vi "ArmControlCalibrate.vi"() -> ()   [LabVIEW 2015]
uses:
  <vilib>/Rock Robotics/WPI/CAN/TalonSRX/WPI_CANTalonSRX_APIFeedbackSelect.ctl
  <vilib>/Rock Robotics/WPI/CAN/TalonSRX/WPI_CANTalonSRX_APIControlMode.ctl
  <vilib>/Rock Robotics/WPI/Joystick/WPI_JoystickDeviceEnum.ctl
  <vilib>/Platform/TimedLoop/XDataNode/timing_clust.ctl
  <vilib>/Platform/TimedLoop/XDataNode/nitl_modes.ctl
  <vilib>/Platform/TimedLoop/XDataNode/wakeup.ctl
  <vilib>/Rock Robotics/WPI/MotorControl/WPI_MotorControlOpenCANTalonSRX.vi
  Team900-VIs/Logitech/F510/F510-X.vi
  <vilib>/addons/control/pid/pid.llb/PID Control Input Filter (DBL).vi
  <vilib>/addons/control/pid/pid.llb/PID (DBL).vi
  Robot Global Data.vi
  <vilib>/Utility/config.llb/Read Key (Double).vi
  <vilib>/Utility/config.llb/Write Key (Double).vi
  <vilib>/Platform/TimedLoop/XDataNode/XDataNode.xnode
  <vilib>/Platform/TimedLoop/XDataNode/XDNodeRunTimeDep.lvlib
  <vilib>/Utility/config.llb/NI_LVConfig.lvlib
  Team900-VIs/Team900SwerveDrive/Team900SwerveDrive.lvlib
  <vilib>/addons/control/pid/NI_PID_pid.lvlib
panel:
  in  "Motor to set offset":enum16{"Pivot", "Wrist", "Claw"}(ring)
  in  "Set":bool
  in  "stop":bool
  in  "Mode":enum32{"Manual Mode", "PID Tuning"}(tab)
  out "(manual) error out":errorcluster
  out "Sensor Position \n(manual) (offset)":dbl
  in  "Control this motor":enum16{"Pivot", "Extension", "Wrist", "Claw"}(ring)
  in  "Max %Vbus":dbl=0.1 format="%#_13g"
  out "Forward Limit Switch Closed":bool
  out "Reverse Limit Switch Closed":bool
  out "Applied Throttle (manual)":dbl
  out "raw sensor position":dbl
  out "Pivot Offset":dbl
  out "Claw Offset (m)":dbl
  out "Wrist Offset":dbl
  out "analog in chart":dbl(graph)
  in  "NI PID":bool
  in  "Setpoint":T1
  in  "Enable":T2
  in  "Motor Controller":enum16{"Pivot", "Extension", "Wrist"}(ring)
  in  "PID":cluster{"P":dbl, "I":dbl, "D":dbl}
  out "error out":errorcluster
  in  "Set":bool=TRUE
  in  "Ramp Rate":dbl
  out "Applied Throttle":dbl
  out "Encoder Position":dbl
  out "Analog In":dbl
  out "Sensor Position":dbl
  out "Difference":dbl
  out "Waveform Chart":cluster{"Pivot":dbl, "Sensor Position":dbl, dbl}(graph)
  out "Angle":dbl(knob) scale=3.14159..-3.14159
  out "Extension":dbl(slide) scale=0.0..100.0
  in  "Claw":bool
  in  "output range":cluster{"output high":dbl, "output low":dbl}={"output high"=100.0, "output low"=-100.0} {"output low" format="%.2f"; "output high" format="%.2f"}
  in  "PID gains":T3={"proportional gain (Kc)"=1.0, "integral time (Ti, min)"=0.0, "derivative time (Td, min)"=0.0} {"derivative time (Td, min)" format="%.3f"; "integral time (Ti, min)" format="%.3f"; "proportional gain (Kc)" format="%.3f"}
  # "360 Ticks on extension"
  # "Left Stick controls whatever motor is selected"
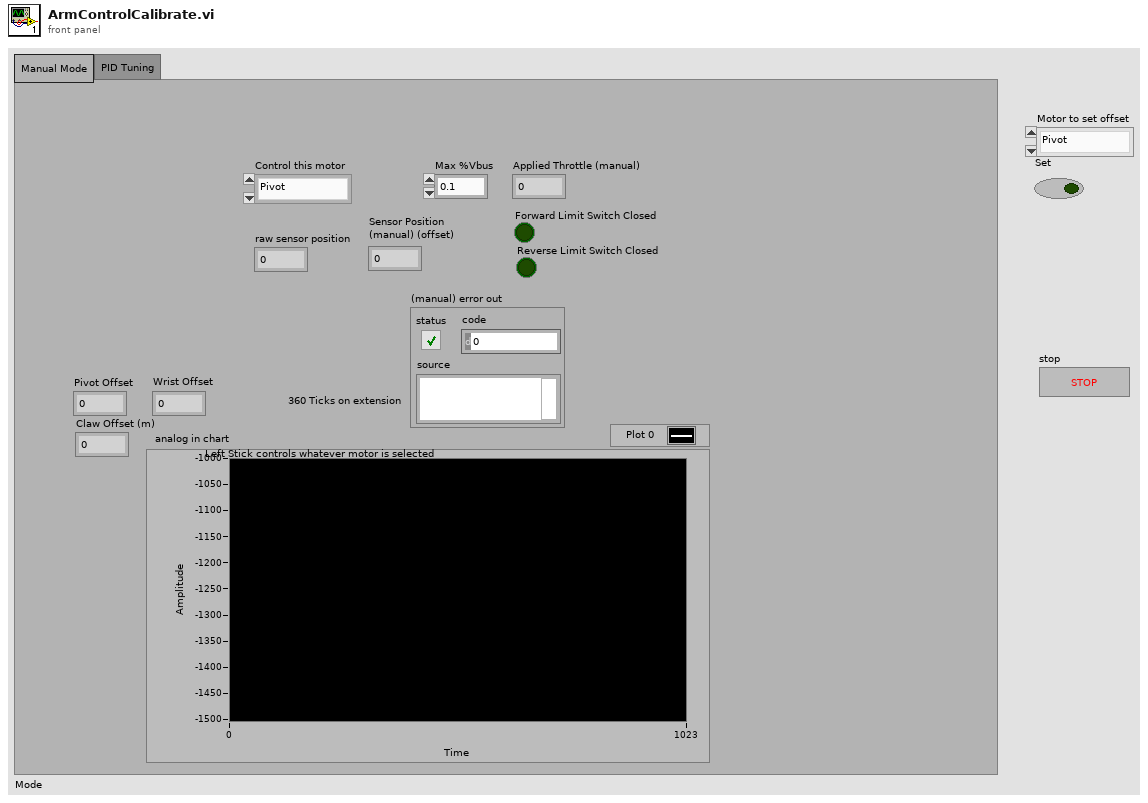
[diagram p1: front panel]
types:
  T1 = cluster{"Pivot":dbl, "Extension":dbl, "Wrist":dbl}
  T2 = cluster{"Pivot":bool, "Exension":bool, "Wrist":bool}
  T3 = cluster{"proportional gain (Kc)":dbl, "integral time (Ti, min)":dbl, "derivative time (Td, min)":dbl}
  T4 = typedef "WPI_CANTalonSRX_APIFeedbackSelect.ctl" = enum16{"Digital Quadrature Encoder", "Analog Potentiometer", "Analog Encoder"}
  T5 = cluster{"Feedback Sensor":T4, "Device Number":u8, "Invert Motor":bool, "Reverse Sensor":bool}
  T6 = typedef "WPI_CANTalonSRX_APIControlMode.ctl" = enum8{"Percent VBus", "Speed", "Position", "Slave", "Unchanged / Invalid"}
  T7 = typedef "NI_LVConfig.lvlib/Config Data RefNum.ctl" = refnum<k1>
  T8 = cluster{"Feedback Sensor":T4, "Device Number":u8, "Invert Motor":bool, "Reverse Sensor":bool}[]
  T9 = typedef "WPI_MotorControlDeviceRef.ctl" = cluster{"DeviceStatus":errorcluster, "Type":T10, "PWM":cluster{"PWM Channel":T11, "DeadBand":T12}, "CAN":cluster{"Device Number":u8, "Control Mode":T13, "Semaphore":T14, "Max Vout":dbl, "TalonSRX Control Mode":T6}, "Invert":bool, "TransformRef":T15, "InvTransformRef":T15}
  T10 = typedef "WPI_MotorControlType.ctl" = enum16{"PWM", "CAN", "CANTalonSRX"}
  T11 = typedef "FPGA_DIOPWMChannel.ctl" = enum8{"PWM 0", "PWM 1", "PWM 2", "PWM 3", "PWM 4", "PWM 5", "PWM 6", "PWM 7", "PWM 8", "PWM 9", "PWM MXP 0", "PWM MXP 1", "PWM MXP 2", "PWM MXP 3", "PWM MXP 4", "PWM MXP 5", "PWM MXP 6", "PWM MXP 7", "PWM MXP 8", "PWM MXP 9", "Invalid"}
  T12 = typedef "WPI_PWMDeadband.ctl" = cluster{"Name":string, "maxPositivePwm":i32, "minPositivePwm":i32, "centerPwm":i32, "maxNegativePwm":i32, "minNegativePwm":i32, "angularRange":u16}
  T13 = typedef "WPI_CANJaguar_ControlMode.ctl" = enum8{"Percent VBus", "Current", "Speed", "Position", "Voltage"}
  T14 = typedef "Semaphore RefNum" = refnum<k1>
  T15 = typedef "WPI_PWMTransform_ConPane.ctl" = refnum<vi>
  T16 = typedef "WPI_CANTalonSRX_GlobalStatus.ctl" = cluster{"Applied Throttle":dbl, "Module Enabled":bool, "CAN Error":errorcluster, "Closed Loop Error":dbl, "Forward Limit Switch Closed":bool, "Reverse Limit Switch Closed":bool, "Sensor Position":dbl, "Sensor Velocity":dbl, "Current":dbl, "Sticky Fault - Over Temp":bool, "Sticky Fault - Under Voltage":bool, "Sticky Fault - Forward Limit":bool, "Sticky Fault - Reverse Limit":bool, "Sticky Fault - Forward Soft Limit":bool, "Sticky Fault - Reverse Soft Limit":bool, "Brake is Enabled":bool, "Encoder Position":dbl, "Encoder Velocity":dbl, "Encoder Index Count":dbl, "Encoder A Pin State":bool, "Encoder B Pin State":bool, "Encoder Index Pin State":bool, "Analog In":dbl, "Analog In Velocity":dbl, "Temperature (C)":dbl, "Battery Voltage":dbl}
  T17 = typedef "WPI_JoystickDeviceEnum.ctl" = enum16{"USB 0", "USB 1", "USB 2", "USB 3", "USB 4", "USB 5"}
  T18 = enum16{"Open", "Close", "Continue", "Stop", "Toggle"}
  T19 = typedef "XDNodeRunTimeDep.lvlib/timing_clust.ctl" = cluster{"Expected End [f-1]":u64, "Actual End [f-1]":u64, "Finished Late? [f-1]":bool, "Expected End [i-1]":u64, "Actual End [i-1]":u64, "Finished Late? [i-1]":bool, "Expected Start [i]":u64, "Actual Start [i]":u64, "Expected Start [f]":u64, "Actual Start [f]":u64, "Source Name":string, "Structure Name":string, "Period":i64, "Deadline":i64, "Offset":i64, "Start":i64, "Priority":i32, "Timeout":i32, "Mode":T20, "Wakeup Reason":T21, "Error":errorcluster, "Source Type":string, "Secondary Source Type":string, "Global End Time":u64, "Global Start Time":u64, "Frame Duration":u64, "Iteration Duration":u64, "Assigned CPU":i32, "I/O Scan Engine Mode":u32}
  T20 = typedef "XDNodeRunTimeDep.lvlib/nitl_modes.ctl" = enum32{"No Change", "Process missed periods, maintain original phase", "Discard missed periods, maintain original phase", "Process missed periods, ignore original phase", "Discard missed periods, ignore original phase"}
  T21 = typedef "XDNodeRunTimeDep.lvlib/wakeup.ctl" = enum32{"Normal", "Aborted", "Asynchronous wakeup", "Timing source error", "Timed loop error", "Timeout"}
  T22 = typedef "WPI_JoystickDevRef.ctl" = cluster{"Device":T17}
  T23 = cluster{"Applied Throttle":dbl, "Encoder Position":dbl, "Sensor Position":dbl, "Analog In":dbl}
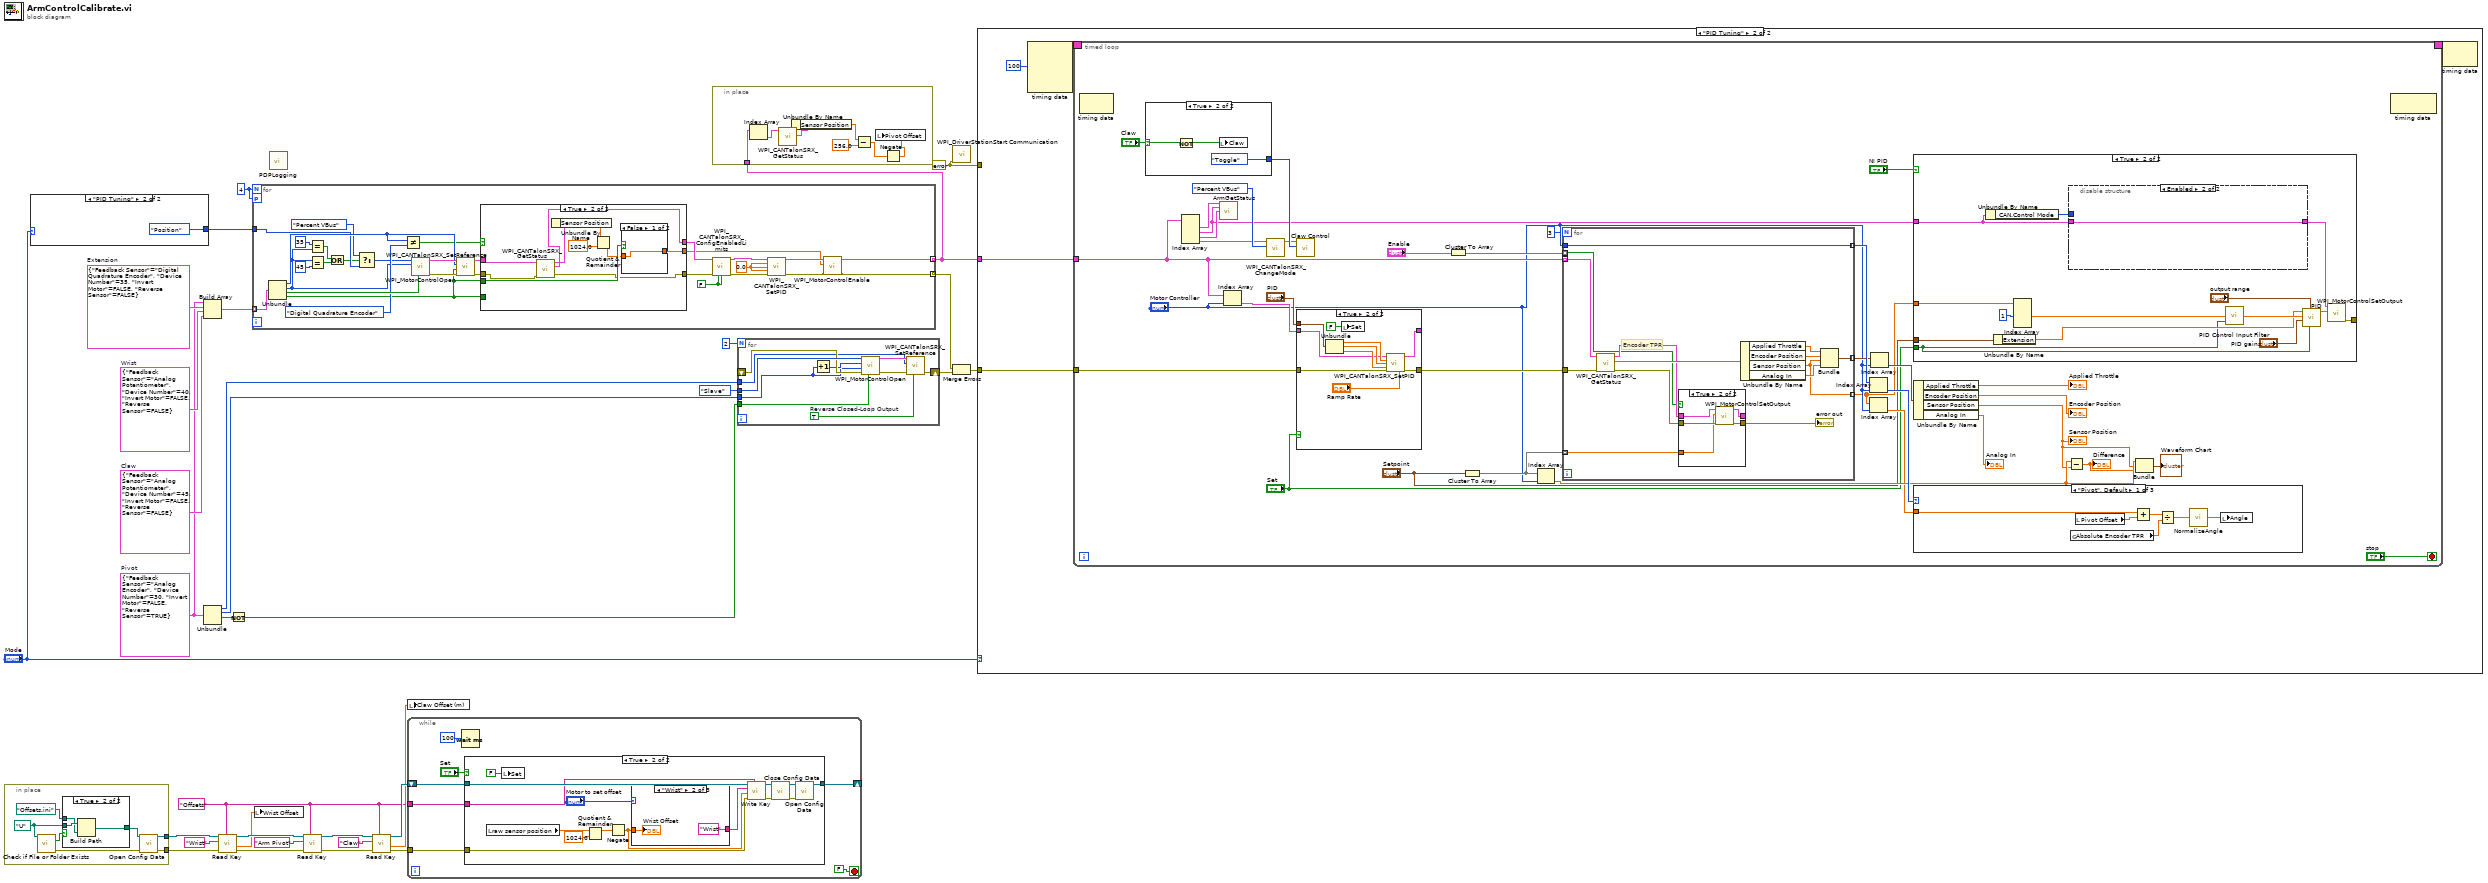
[diagram p0: block diagram]
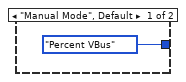
[diagram p2: hidden frame]
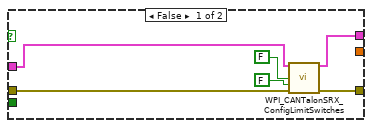
[diagram p3: hidden frame]
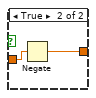
[diagram p4: hidden frame]
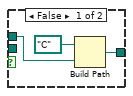
[diagram p5: hidden frame]
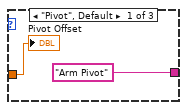
[diagram p7: hidden frame]
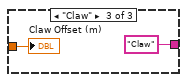
[diagram p8: hidden frame]
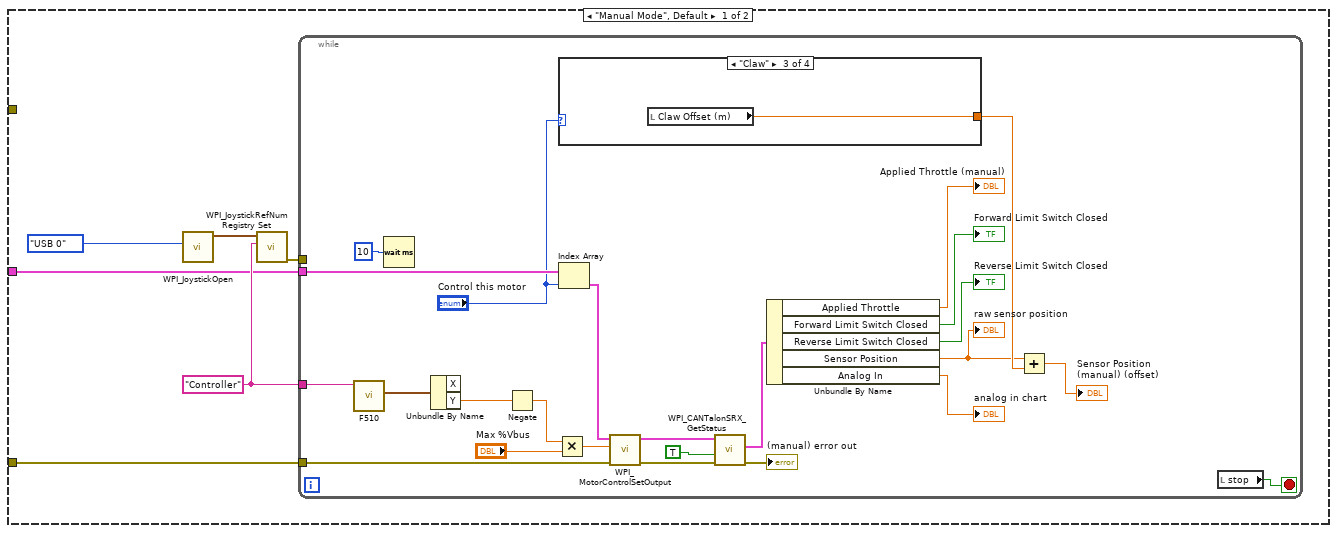
[diagram p9: hidden frame]
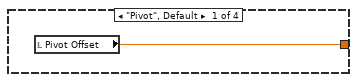
[diagram p10: hidden frame]
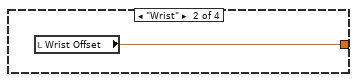
[diagram p11: hidden frame]
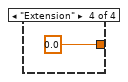
[diagram p12: hidden frame]
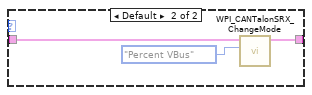
[diagram p15: hidden frame]
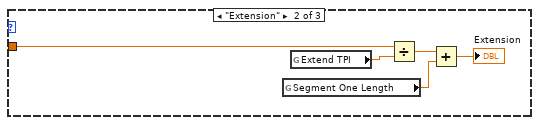
[diagram p16: hidden frame]
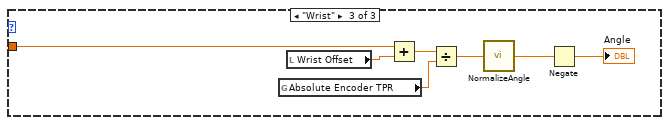
[diagram p17: hidden frame]
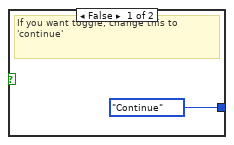
[diagram p19: hidden frame]
diagram:
  w2 = T5 {"Feedback Sensor"=enum."Analog Encoder", "Device Number"=30, "Invert Motor"=FALSE, "Reverse Sensor"=TRUE}  # Pivot
  w3 = T5 {"Feedback Sensor"=enum."Digital Quadrature Encoder", "Device Number"=35, "Invert Motor"=FALSE, "Reverse Sensor"=FALSE}  # Extension
  w16 = 4
  w19 = "Offsets" ("section")
  w17 = T5 {"Feedback Sensor"=enum."Analog Potentiometer", "Device Number"=45, "Invert Motor"=FALSE, "Reverse Sensor"=FALSE}  # Claw
  w18 = T5 {"Feedback Sensor"=enum."Analog Potentiometer", "Device Number"=40, "Invert Motor"=FALSE, "Reverse Sensor"=FALSE}  # Wrist
  w33 = errorcluster {"status"=FALSE, "code"=0, "source"=""} ("error constant")
  n1 = in-place {
    in-place-border: [w39] -> w32
    in-place-border: [w38] -> w31
    w34 = path "U:/" ("base path")
    n2 = call <vilib>:"Check if File or Folder Exists.vi"("path"=w34) -> ("error out"=w40:errorcluster, "file or folder exists?"=w35:bool)  [unwired: 8 in, 1 out]
    n3 = case shown="True" w35 {
      tunnel: path "Offsets.ini" ("default name") -> [w43 w44]
      tunnel: [w42 w45] -> w37
      tunnel: w34 -> [_ w46]
      frame False {
        n4 = Build Path(base path=path "C:/", name or relative path=w43) -> (appended path=w42:path)
      }
      frame True {
        n5 = Build Path(base path=w46, name or relative path=w44) -> (appended path=w45:path)
      }
    }
    n6 = call <vilib>:"Open Config Data.vi"("error in (no error)"=w40, "configuration file path"=w37) -> ("error out"=w39:errorcluster, "refnum"=w38:T7)  [unwired: 1 in, 7 out]
  }
  n7 = case shown="\"PID Tuning\"" "Mode" {
    tunnel: [WPI_CANTalonSRX_APIControlMode."Percent VBus" ("Control Mode") WPI_CANTalonSRX_APIControlMode."Position" ("Control Mode")] -> w12
    frame "Manual Mode", Default {
    }
    frame "PID Tuning" {
    }
  }
  n8 = Build Array(w2, w3, w18, w17) -> (w15:T8)
  n9 = Unbundle(w2) -> ("Feedback Sensor"=w8:T4, "Device Number"=w9:u8, "Invert Motor"=w6:bool)  [unwired: 1 out]
  n10 = call-poly <vilib>:"Read Key.vi"("section"=w19, "error in (no error)"=w32, "key"="Wrist", "refnum"=w31) -> ("error out"=w27:errorcluster, "value"=w21:dbl, "refnum out"=w30:T7)  [unwired: 4 in, 1 out]
  n11 = Not(x=w6) -> (.not. x?=w7:bool)
  n12 = for {
    N: w16 -> [_]
    workers-P: w16 -> [_]
    tunnel: [w51] -> w1 mode=indexing
    tunnel: [w52] -> w14 mode=indexing
    tunnel: w15 -> [w76] mode=indexing
    tunnel: w12 -> [w66]
    w55 = FALSE
    w70 = 0.0
    n13 = Unbundle(w76) -> ("Feedback Sensor"=w72:T4, "Device Number"=w62:u8, "Invert Motor"=w75:bool, "Reverse Sensor"=w50:bool)
    n14 = Equal?(x=u8 35, y=w62) -> (x = y?=w64:bool)
    n15 = Equal?(x=w62, y=u8 45) -> (x = y?=w63:bool)
    n16 = Or(x=w64, y=w63) -> (x .or. y?=w65:bool)
    n17 = Select(t=WPI_CANTalonSRX_APIControlMode."Percent VBus" ("f"), s=w65, f=w66) -> (s? t:f=w68:T6)
    n18 = Not Equal?(x=w72, y=WPI_CANTalonSRX_APIFeedbackSelect."Digital Quadrature Encoder") -> (x != y?=w69:bool)
    n19 = call-poly <vilib>:"WPI_MotorControlOpen.vi"("Invert"=w75, "Device Number"=w62, "Control Mode"=w68) -> ("error out"=w78:errorcluster, "MotorControlDeviceRef"=w77:T9)  [unwired: 7 in]
    n20 = call <vilib>:"WPI_CANTalonSRX_SetReference.vi"("error in (no error)"=w78, "Reverse Feedback Sensor"=w50, "Feedback Reference"=w72, "CAN Talon SRX Ref"=w77) -> ("error out"=w74:errorcluster, "CAN Talon SRX Ref"=w73:T9)  [unwired: 6 in]
    n21 = case shown="True" w69 {
      tunnel: w50 -> [_ _]
      tunnel: w74 -> [w79 w92]
      tunnel: w73 -> [w80 w93]
      tunnel: [w84 w88] -> w59
      tunnel: [w83 w87] -> w58
      tunnel: w50 -> [_ w91]
      tunnel: [_ w89] -> w49
      frame False {
        n22 = call <vilib>:"WPI_CANTalonSRX_ConfigLimitSwitches.vi"("CAN Talon SRX Ref"=w80, "Forward Limit Switch Normally Open"=FALSE, "Reverse Limit Switch Normally Open"=FALSE, "error in (no error)"=w79) -> ("CAN Talon SRX Ref"=w84:T9, "error out"=w83:errorcluster)  [unwired: 10 in]
      }
      frame True {
        n23 = call <vilib>:"WPI_CANTalonSRX_GetStatus.vi"("error in (no error)"=w92, "CAN Talon SRX Ref"=w93) -> ("error out"=w87:errorcluster, "Talon SRX Status"=w94:T16, "CAN Talon SRX Ref"=w88:T9)  [unwired: 7 in]
        n24 = Unbundle By Name(w94) -> ("Sensor Position"=w90:dbl)
        n25 = Quotient & Remainder(x=w90, y=1024.0) -> (floor(x/y)=w86:dbl)  [unwired: 1 out]
        n26 = case shown="False" w91 {
          tunnel: w86 -> [w95 w97]
          tunnel: [w95 w96] -> w89
          frame False {
          }
          frame True {
            n27 = Negate(x=w97) -> (-x=w96:dbl)
          }
        }
      }
    }
    n28 = call <vilib>:"WPI_CANTalonSRX_ConfigEnabledLimits.vi"("CAN Talon SRX Ref"=w59, "error in (no error)"=w58, "Forward Soft Limit Enable"=w55, "Reverse Soft Limit Enable"=w55) -> ("CAN Talon SRX Ref"=w57:T9, "error out"=w56:errorcluster)  [unwired: 10 in]
    n29 = call <vilib>:"WPI_CANTalonSRX_SetPID.vi"("CAN Talon SRX Ref"=w57, "P"=w70, "I"=w70, "D"=w70, "error in (no error)"=w56) -> ("CAN Talon SRX Ref Out"=w54:T9, "error out"=w53:errorcluster)  [unwired: 9 in]
    n30 = call <vilib>:"WPI_MotorControlEnable.vi"("error in (no error)"=w53, "Encoder Initial Position"=w49, "CAN Jaguar Ref"=w54) -> ("error out"=w52:errorcluster, "CAN Jaguar Ref"=w51:T9)  [unwired: 7 in]
  }
  n31 = local write "Wrist Offset"(w21) -> ()
  n32 = call "PDPLogging.vi"() -> ()  [unwired: 12 in]
  n33 = call-poly <vilib>:"Read Key.vi"("section"=w19, "error in (no error)"=w27, "key"="Arm Pivot", "refnum"=w30) -> ("error out"=w26:errorcluster, "refnum out"=w29:T7)  [unwired: 4 in, 2 out]
  n34 = call-poly <vilib>:"Read Key.vi"("section"=w19, "error in (no error)"=w26, "key"="Claw", "refnum"=w29) -> ("error out"=w25:errorcluster, "value"=w20:dbl, "refnum out"=w28:T7)  [unwired: 4 in, 1 out]
  n35 = local write "Claw Offset (m)"(w20) -> ()
  n36 = while {
    tunnel: w25 -> [w103]
    shift-right: [w99] -> _
    shift-left: w28 -> [w104]
    tunnel: w19 -> [w98]
    stop <- FALSE stop-if-true
    n37 = Wait (ms)(milliseconds to wait=u32 100) -> ()  [unwired: 1 out]
    n38 = case shown="True" "Set" {
      tunnel: w104 -> [w105 w120]
      tunnel: w103 -> [_ w119]
      tunnel: [w105 w110] -> w99
      tunnel: w98 -> [_ w106]
      frame False {
      }
      frame True {
        n39 = local read "raw sensor position"() -> (w115:dbl)
        n40 = local write "Set"(FALSE ("Zero Position")) -> ()
        n41 = Quotient & Remainder(x=w115, y=1024.0) -> (x-y*floor(x/y)=w116:dbl)  [unwired: 1 out]
        n42 = Negate(x=w116) -> (-x=w107:dbl)
        n43 = case shown="\"Wrist\"" "Motor to set offset" {
          tunnel: ["Arm Pivot" "Wrist" "Claw"] -> w108
          tunnel: w107 -> [w121 w123 w125]
          frame "Pivot", Default {
            "Pivot Offset" <- w121
          }
          frame "Wrist" {
            "Wrist Offset" <- w123
          }
          frame "Claw" {
            "Claw Offset (m)" <- w125
          }
        }
        n44 = call-poly <vilib>:"Write Key.vi"("section"=w106, "error in (no error)"=w119, "value"=w107, "key"=w108, "refnum"=w120) -> ("error out"=w113:errorcluster, "refnum out"=w114:T7)  [unwired: 4 in, 1 out]
        n45 = call <vilib>:"Close Config Data.vi"("error in (no error)"=w113, "refnum"=w114) -> ("error out"=w111:errorcluster, "file path"=w112:path)  [unwired: 8 in]
        n46 = call <vilib>:"Open Config Data.vi"("error in (no error)"=w111, "configuration file path"=w112) -> ("refnum"=w110:T7)  [unwired: 1 in, 8 out]
      }
    }
  }
  n47 = in-place {
    in-place-border: w1 -> [w133]
    n48 = Index Array(array=w133) -> (element=w132:T9)  [unwired: 1 in]
    n49 = call <vilib>:"WPI_CANTalonSRX_GetStatus.vi"("CAN Talon SRX Ref"=w132) -> ("Talon SRX Status"=w131:T16)  [unwired: 8 in, 2 out]
    n50 = Unbundle By Name(w131) -> ("Sensor Position"=w130:dbl)
    n51 = Subtract(x=w130, y=256.0) -> (x-y=w128:dbl)
    n52 = Negate(x=w128) -> (-x=w127:dbl)
    n53 = local write "Pivot Offset"(w127) -> ()
  }
  n54 = for {
    N: 2 -> [_]
    tunnel: WPI_CANTalonSRX_APIControlMode."Slave" ("Control Mode") -> [w143]
    tunnel: w9 -> [w135]
    tunnel: w7 -> [w142]
    shift-right: [w138] -> w4
    shift-left: _ -> [w141]
    tunnel: w8 -> [w137]
    w134 = TRUE  # Reverse Closed-Loop Output
    n55 = Increment(x=w135) -> (x+1=w136:u8)
    n56 = call-poly <vilib>:"WPI_MotorControlOpen.vi"("Invert"=w142, "error in (no error)"=w141, "Master Device Number"=w135, "Device Number"=w136, "Control Mode"=w143) -> ("error out"=w139:errorcluster, "MotorControlDeviceRef"=w140:T9)  [unwired: 5 in]
    n57 = call <vilib>:"WPI_CANTalonSRX_SetReference.vi"("Reverse Closed-Loop Output"=w134, "error in (no error)"=w139, "Feedback Reference"=w137, "CAN Talon SRX Ref"=w140) -> ("error out"=w138:errorcluster)  [unwired: 6 in, 1 out]
  }
  n58 = call <vilib>:"WPI_DriverStationStart Communication.vi"("error in (no error)"=w33) -> ()  [unwired: 11 in]
  n59 = Merge Errors(w14, w4) -> (w5:errorcluster)
  n60 = case shown="\"PID Tuning\"" "Mode" {
    tunnel: w33 -> [_ _]
    tunnel: w1 -> [w145 w180]
    tunnel: w5 -> [w144 w179]
    frame "Manual Mode", Default {
      w147 = "Controller" ("refnum name")
      n61 = call <vilib>:"WPI_JoystickOpen.vi"("JoystickDevice"=WPI_JoystickDeviceEnum."USB 0") -> ("JoystickDevRef"=w149:T22)  [unwired: 10 in]
      n62 = call <vilib>:"WPI_JoystickRefNum Registry Set.vi"("refnum name"=w147, "JoystickDevRef"=w149) -> ("error out"=w146:errorcluster)  [unwired: 8 in, 1 out]
      n63 = while {
        tunnel: w145 -> [w172]
        tunnel: w144 -> [w150]
        tunnel: w147 -> [w171]
        tunnel: w146 -> [_]
        stop <- w166 stop-if-true
        n64 = call-poly "F510.vi"("refnum name"=w171) -> ("Left Stick"=w170:cluster{"X":dbl, "Y":dbl})  [unwired: 4 in, 6 out]
        n65 = Wait (ms)(milliseconds to wait=u32 10) -> ()  [unwired: 1 out]
        n66 = Unbundle By Name(w170) -> ("Y"=w169:dbl)  [unwired: 1 out]
        n67 = Negate(x=w169) -> (-x=w161:dbl)
        n68 = Multiply(x=w161, y="Max %Vbus") -> (x*y=w167:dbl)
        n69 = case shown="\"Claw\"" "Control this motor" {
          tunnel: [w174 w175 w176 0.0] -> w154
          frame "Pivot", Default {
            n70 = local read "Pivot Offset"() -> (w174:dbl)
          }
          frame "Wrist" {
            n71 = local read "Wrist Offset"() -> (w175:dbl)
          }
          frame "Claw" {
            n72 = local read "Claw Offset (m)"() -> (w176:dbl)
          }
          frame "Extension" {
          }
        }
        n73 = Index Array(array=w172, index="Control this motor") -> (element=w162:T9)
        n74 = call <vilib>:"WPI_MotorControlSetOutput.vi"("error in (no error)"=w150, "Output"=w167, "MotorControlDevRef"=w162) -> ("error out"=w165:errorcluster, "MotorControlDevRef"=w164:T9)  [unwired: 6 in, 1 out]
        n75 = call <vilib>:"WPI_CANTalonSRX_GetStatus.vi"("error in (no error)"=w165, "Clear Sticky Faults"=TRUE, "CAN Talon SRX Ref"=w164) -> ("error out"=→"(manual) error out":errorcluster, "Talon SRX Status"=w163:T16)  [unwired: 6 in, 1 out]
        n76 = Unbundle By Name(w163) -> ("Applied Throttle"=→"Applied Throttle (manual)":dbl, "Forward Limit Switch Closed"=→"Forward Limit Switch Closed":bool, "Reverse Limit Switch Closed"=→"Reverse Limit Switch Closed":bool, "Sensor Position"=w153:dbl, "Analog In"=→"analog in chart":dbl)
        "raw sensor position" <- w153
        n77 = Add(x=w153, y=w154) -> (x+y=→"Sensor Position \n(manual) (offset)":dbl)
        n78 = local read "stop"() -> (w166:bool)
      }
    }
    frame "PID Tuning" {
      n79 = node-c288(i64 100 ("Period")) -> (w182:T19)  [unwired: 3 in]
      n80 = timed-loop {
        timing: w182 -> [_]
        timing-out: [_] -> w181
        tunnel: w180 -> [w208]
        tunnel: w179 -> [w213]
        stop <- "stop" stop-if-true
        n81 = node-c288() -> ()  [unwired: 1 in, 1 out]
        n82 = case shown="True" "Claw" {
          selector: "Claw" -> [_ w281]
          tunnel: [T18."Continue" ("Operation") T18."Toggle" ("Operation")] -> w212
          frame False {
            # "If you want toggle, change this to 'continue'"
          }
          frame True {
            n83 = Not(x=w281) -> (.not. x?=w280:bool)
            n84 = local write "Claw"(w280) -> ()
          }
        }
        n85 = Index Array(array=w208) -> (element #1=w193:T9, element #2=w186:T9, element #3=w192:T9, element #4=w191:T9)  [unwired: 4 in]
        n86 = call "ArmGetStatus.vi"("Pivot Ref"=w193, "ExtensionRef"=w186, "Wrist Ref"=w192) -> ()  [unwired: 4 in, 9 out]
        n87 = Index Array(array=w208, index="Motor Controller") -> (element=w214:T9)
        n88 = call <vilib>:"WPI_CANTalonSRX_ChangeMode.vi"("Control Mode"=WPI_CANTalonSRX_APIControlMode."Percent VBus", "CAN Talon SRX Ref"=w191) -> ("CAN Talon SRX Ref"=w209:T9)  [unwired: 8 in, 1 out]
        n89 = call "Claw Control.vi"("Operation"=w212, "MotorControlDevRef"=w209) -> ()  [unwired: 4 in, 4 out]
        n90 = case shown="True" "Set" {
          tunnel: "PID" -> [_ w291]
          tunnel: w214 -> [w284 w290]
          tunnel: [w284 w288] -> _
          tunnel: [w283 w287] -> w215
          tunnel: w213 -> [w283 w285]
          frame False {
          }
          frame True {
            n91 = Unbundle(w291) -> ("P"=w292:dbl, "I"=w293:dbl, "D"=w294:dbl)
            n92 = local write "Set"(FALSE) -> ()
            n93 = call <vilib>:"WPI_CANTalonSRX_SetPID.vi"("CAN Talon SRX Ref"=w290, "P"=w292, "I"=w293, "D"=w294, "error in (no error)"=w285, "Ramp Rate"="Ramp Rate") -> ("CAN Talon SRX Ref Out"=w288:T9, "error out"=w287:errorcluster)  [unwired: 8 in]
          }
        }
        n94 = Cluster To Array(cluster="Enable") -> (array=w203:bool[])
        n95 = Cluster To Array(cluster="Setpoint") -> (array=w200:dbl[])
        n96 = Index Array(array=w200, index="Motor Controller") -> (element=w201:dbl)
        n97 = for {
          N: 3 -> [_]
          tunnel: w208 -> [w270] mode=indexing
          tunnel: w215 -> [w268]
          tunnel: "Motor Controller" -> [w265]
          tunnel: [w265] -> w207 mode=indexing
          tunnel: [w258] -> w185 mode=indexing
          tunnel: [w262] -> w204 mode=indexing
          tunnel: w200 -> [w260] mode=indexing
          tunnel: w203 -> [w259] mode=indexing
          # "Encoder TPR"
          n98 = call <vilib>:"WPI_CANTalonSRX_GetStatus.vi"("error in (no error)"=w268, "CAN Talon SRX Ref"=w270) -> ("error out"=w266:errorcluster, "Talon SRX Status"=w269:T16, "CAN Talon SRX Ref"=w267:T9)  [unwired: 7 in]
          n99 = case shown="True" w259 {
            tunnel: w267 -> [w272 w278]
            tunnel: w266 -> [w273 w277]
            tunnel: [w273 w276] -> w271
            tunnel: [w272 w275] -> _
            tunnel: w260 -> [_ w274]
            frame False {
            }
            frame True {
              n100 = call <vilib>:"WPI_MotorControlSetOutput.vi"("error in (no error)"=w277, "Output"=w274, "MotorControlDevRef"=w278) -> ("error out"=w276:errorcluster, "MotorControlDevRef"=w275:T9)  [unwired: 6 in, 1 out]
            }
          }
          "error out" <- w271
          n101 = Unbundle By Name(w269) -> ("Applied Throttle"=w264:dbl, "Encoder Position"=w263:dbl, "Sensor Position"=w258:dbl, "Analog In"=w261:dbl)
          n102 = Bundle("Applied Throttle"=w264, "Encoder Position"=w263, "Sensor Position"=w258, "Analog In"=w261) -> (w262:T23)  [unwired: 1 in]
        }
        n103 = Index Array(array=w207, index="Motor Controller") -> (element=w206:enum16{"Pivot", "Extension", "Wrist"})
        n104 = Index Array(array=w185, index="Motor Controller") -> (element=w196:dbl)
        n105 = Index Array(array=w204, index="Motor Controller") -> (element=w205:T23)
        n106 = case shown="True" "NI PID" {
          tunnel: w186 -> [_ w230]
          tunnel: w185 -> [_ w228]
          tunnel: "Setpoint" -> [_ w224]
          tunnel: [_ w219] -> _
          tunnel: "Set" -> [_ w218]
          frame False {
          }
          frame True {
            n107 = Unbundle By Name(w230) -> ("CAN.Control Mode"=w231:T13)
            n108 = Unbundle By Name(w224) -> ("Extension"=w223:dbl)
            n109 = Index Array(array=w228, index #2=1 ("index")) -> (element #2=w221:dbl)  [unwired: 3 in, 3 out]
            n110 = disable-structure shown="Enabled" {
              disable-tunnel: w231 -> [w234 _]
              disable-tunnel: w230 -> [w233 w239]
              disable-tunnel: [w232 w239] -> w229
              frame Disabled {
                n111 = case shown="\"Percent VBus\"" w234 {
                  tunnel: w233 -> [w235 w237]
                  tunnel: [w235 w236] -> w232
                  frame "Percent VBus" {
                  }
                  frame Default {
                    n112 = call <vilib>:"WPI_CANTalonSRX_ChangeMode.vi"("Control Mode"=WPI_CANTalonSRX_APIControlMode."Percent VBus", "CAN Talon SRX Ref"=w237) -> ("CAN Talon SRX Ref"=w236:T9)  [unwired: 8 in, 1 out]
                  }
                }
              }
              frame Enabled {
              }
            }
            n113 = call-poly <vilib>:"PID Control Input Filter.vi"("reinitialize? (F)"=w218, "input"=w221) -> ("output"=w227:dbl)  [unwired: 3 in]
            n114 = call-poly <vilib>:"PID.vi"("reinitialize? (F)"=w218, "output range"="output range", "PID gains"="PID gains", "process variable"=w227, "setpoint"=w223) -> ("output"=w222:dbl)  [unwired: 5 in, 1 out]
            n115 = call <vilib>:"WPI_MotorControlSetOutput.vi"("Output"=w222, "MotorControlDevRef"=w229) -> ("error out"=w219:errorcluster)  [unwired: 7 in, 2 out]
          }
        }
        n116 = Unbundle By Name(w205) -> ("Applied Throttle"=→"Applied Throttle":dbl, "Encoder Position"=→"Encoder Position":dbl, "Sensor Position"=w195:dbl, "Analog In"=→"Analog In":dbl)
        "Sensor Position" <- w195
        n117 = case shown="\"Pivot\", Default" w206 {
          tunnel: w196 -> [w241 w248 w253]
          frame "Pivot", Default {
            n118 = global read "Robot Global Data.vi" "Absolute Encoder TPR"() -> (w242:dbl)
            n119 = local read "Pivot Offset"() -> (w245:dbl)
            n120 = Add(x=w241, y=w245) -> (x+y=w244:dbl)
            n121 = Divide(x=w244, y=w242) -> (x/y=w243:dbl)
            n122 = call "NormalizeAngle.vi"("angle (rad)"=w243) -> ("angle (between pi and -pi)"=w240:dbl)
            n123 = local write "Angle"(w240) -> ()
          }
          frame "Extension" {
            n124 = global read "Robot Global Data.vi" "Segment One Length"() -> (w249:dbl)
            n125 = global read "Robot Global Data.vi" "Extend TPI"() -> (w246:dbl)
            n126 = Divide(x=w248, y=w246) -> (x/y=w247:dbl)
            n127 = Add(x=w247, y=w249) -> (x+y=→"Extension":dbl)
          }
          frame "Wrist" {
            n128 = global read "Robot Global Data.vi" "Absolute Encoder TPR"() -> (w254:dbl)
            n129 = local read "Wrist Offset"() -> (w256:dbl)
            n130 = Add(x=w253, y=w256) -> (x+y=w257:dbl)
            n131 = Divide(x=w257, y=w254) -> (x/y=w255:dbl)
            n132 = call "NormalizeAngle.vi"("angle (rad)"=w255) -> ("angle (between pi and -pi)"=w251:dbl)
            n133 = Negate(x=w251) -> (-x=→"Angle":dbl)
          }
        }
        n134 = Subtract(x=w201, y=w195) -> (x-y=w188:dbl)
        "Difference" <- w188
        n135 = Bundle("Pivot"=w201, "Sensor Position"=w195, w188) -> (→"Waveform Chart":cluster{"Pivot":dbl, "Sensor Position":dbl, dbl})  [unwired: 1 in]
        n136 = node-c288() -> ()  [unwired: 1 in, 1 out]
      }
      n137 = node-c288(w181) -> ()  [unwired: 1 out]
    }
  }
